vi "Set Value.vi"(8 "error in (no error)":errorcluster, 10 "Value":variant, 11 "Ctrl Reference's in":refnum<class "Ctrl Reference's.lvclass">) -> (0 "error out":errorcluster, 3 "Ctrl Reference's out":refnum<class "Ctrl Reference's.lvclass">, 4 "Ctl Refnum":refnum<vi>)   [LabVIEW 2023, in "Ctrl Reference's.lvclass"]
uses:
  Ctrl Reference's.lvclass
  Ctrl Reference's.lvclass/Ctrl Reference's.ctl
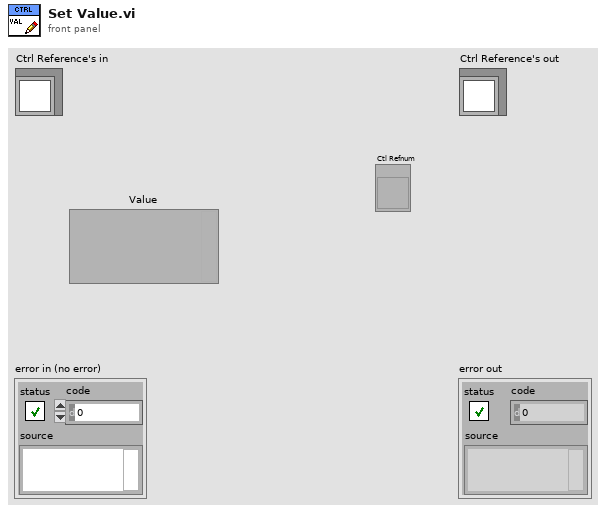
[diagram p1: front panel]
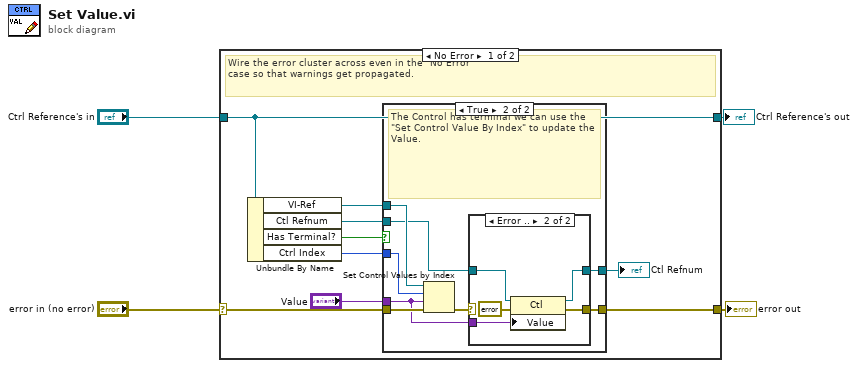
[diagram p0: block diagram]
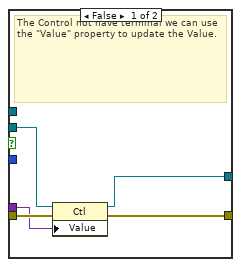
[diagram p2: hidden frame]
diagram:
  n1 = case shown="No Error" "error in (no error)" {
    selector: "error in (no error)" -> [w10 w35]
    tunnel: [w11 w35] -> w3
    tunnel: [w13 w34] -> w1
    tunnel: "Ctrl Reference's in" -> [w13 w34]
    frame No Error {
      # "Wire the error cluster across even in the \"No Error\"\ncase so that warnings get propagated."
      n2 = Unbundle By Name(w13) -> ("VI-Ref"=w8:refnum<vi>, "Ctl Refnum"=w7:refnum<vi>, "Has Terminal?"=w12:bool, "Ctrl Index"=w9:i32)
      n3 = case shown="True" w12 {
        tunnel: [w15 w22] -> w11
        tunnel: w10 -> [w17 w25]
        tunnel: w9 -> [_ w24]
        tunnel: w8 -> [_ w26]
        tunnel: w7 -> [w18 w21]
        tunnel: "Value" -> [w16 w20]
        tunnel: [w14 w19] -> w5
        frame False {
          # "The Control not have terminal we can use the \"Value\" property to update the Value."
          n4 = property class="Ctl"(reference=w18, error in=w17, "Value"=w16) -> (reference out=w14:refnum<vi>, error out=w15:errorcluster)
        }
        frame True {
          # "The Control has terminal we can use the \"Set Control Value By Index\" to update the Value."
          n5 = Set Control Values by Index(0:w26, 1:w24, 2:w20, 3:w25) -> (11:w23:errorcluster)
          n6 = case shown="Error .." w23 {
            selector: w23 -> [w28 _]
            tunnel: [w28 w33] -> w22
            tunnel: w21 -> [w27 w32]
            tunnel: w20 -> [_ w31]
            tunnel: [w27 w30] -> w19
            frame No Error {
            }
            frame Error {
              n7 = property class="Ctl"(reference=w32, error in=errorcluster {"status"=FALSE, "code"=0, "source"=""} ("error in (no error)"), "Value"=w31) -> (reference out=w30:refnum<vi>, error out=w33:errorcluster)
            }
          }
        }
      }
      "Ctl Refnum" <- w5
    }
    frame Error {
    }
  }
  "error out" <- w3
  "Ctrl Reference's out" <- w1
